vi "Read Spectrum Configuration.vi"(8 "error in (no error)":errorcluster, 11 "Red Pitaya Transceiver Driver in":refnum<class "Red Pitaya Transceiver Driver.lvclass">) -> (0 "error out":errorcluster, 2 "Configuration":T1={"Start frequency"=500000.0, "End frequency"=2000000.0, "Coarse step"=40.0, "Step duration"=0.004, "Red Pitaya address"="192.168.1.100", "Open plot \non start"=FALSE, "Fine region centers"=[], "Regions width"=0.0, "Fine step"=1.0} {"Fine step" min=1.0 format="%#_6pHz"; "Regions width" format="%#_6pHz"; "Fine region centers" format="%#_6pHz"; "Step duration" format="%#_6ps"; "Coarse step" format="%#_6pHz"; "End frequency" format="%#_6pHz"; "Start frequency" format="%#_6pHz"}, 3 "Red Pitaya Transceiver Driver out":refnum<class "Red Pitaya Transceiver Driver.lvclass">)   [LabVIEW 2016, in "Red Pitaya Transceiver Driver.lvclass"]
uses:
  Red Pitaya Transceiver Driver.lvclass
  C:/Github/NHMFL_Core/Libraries/Instruments/Instrument Driver/Instrument Driver.lvclass
  Spectrum Configuration.ctl
  Instruments/Instrument Driver/Read User configuration.vi
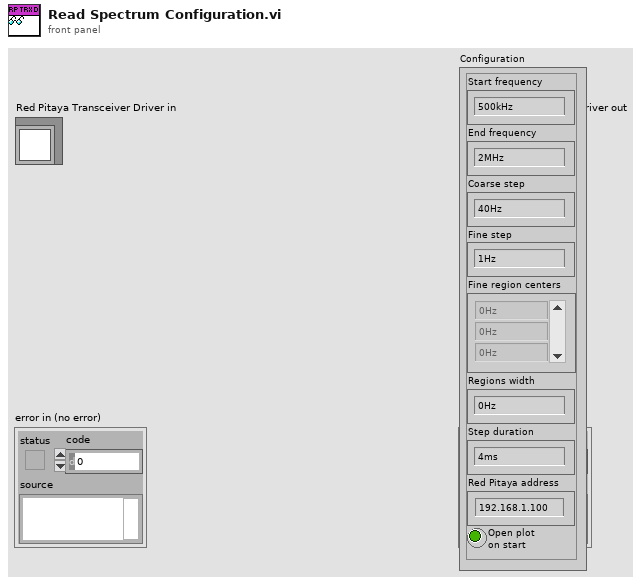
[diagram p1: front panel]
types:
  T1 = typedef "Spectrum Configuration.ctl" = cluster{"Start frequency":dbl, "End frequency":dbl, "Coarse step":dbl, "Step duration":dbl, "Red Pitaya address":string, "Open plot \non start":bool, "Fine region centers":dbl[], "Regions width":dbl, "Fine step":dbl}
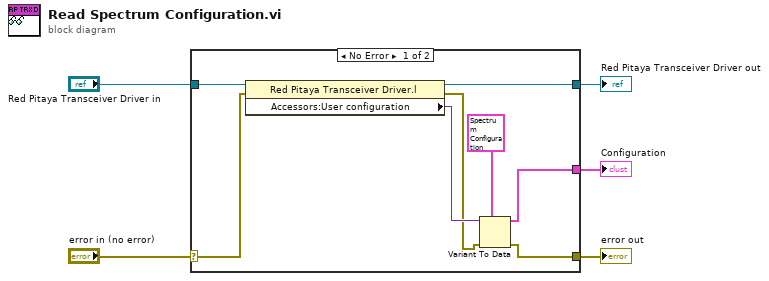
[diagram p0: block diagram]
diagram:
  n1 = case shown="No Error" "error in (no error)" {
    selector: "error in (no error)" -> [w6 w14]
    tunnel: [w10 w14] -> w4
    tunnel: [w9 w15] -> w2
    tunnel: "Red Pitaya Transceiver Driver in" -> [w13 w15]
    tunnel: [w11 _] -> w1
    frame No Error {
      n2 = property class="Red Pitaya Transceiver Driver.l"(reference=w13, error in=w6) -> (reference out=w9:refnum<class "Red Pitaya Transceiver Driver.lvclass">, error out=w7:errorcluster, "Accessors:User configuration"=w8:variant)
      n3 = Variant To Data(error in=w7, type=T1 {"Start frequency"=500000.0, "End frequency"=2000000.0, "Coarse step"=40.0, "Step duration"=0.004, "Red Pitaya address"="192.168.1.100", "Open plot \non start"=FALSE, "Fine region centers"=[], "Regions width"=0.0, "Fine step"=1.0} ("Configuration"), Variant=w8) -> (data=w11:T1, error out=w10:errorcluster)
    }
    frame Error {
    }
  }
  "error out" <- w4
  "Red Pitaya Transceiver Driver out" <- w2
  "Configuration" <- w1
